vi "Get Config.vi"(0 "Sequence path":path=path "C:/ModisEdge/Scope/Test Sequence/ModisEdge.ini", 7 "File":string="ModisEdge.ini") -> (1 "Headers Path":path=path "C:/ModisEdge/Scope/Test Sequence/Headers_ModisEdge.ini", 2 "FixtureID":string="MEScope_Fixture1", 3 "StopTestOnFailure":bool=TRUE, 4 "StationID":string="TSNAFT202", 6 "Test Report Path":path=path "C:/Snap-On/ModisEdge_Scope", 8 "DAQ DEVICE NAME":string="Dev5", 10 "WriteTheHeaders":bool, 14 "UUT_COM":u32=5, 15 "error out":errorcluster)   [LabVIEW 2015]
uses:
  <vilib>/Utility/config.llb/Read Key (Boolean).vi
  <vilib>/Utility/config.llb/Read Key (String).vi
  <vilib>/Utility/config.llb/Read Key (Path).vi
  <vilib>/Utility/config.llb/Read Key (U32).vi
  <vilib>/Utility/config.llb/NI_LVConfig.lvlib
panel:
  out "appended path":path=path "C:/ModisEdge/Scope/Test Sequence/ModisEdge.ini"
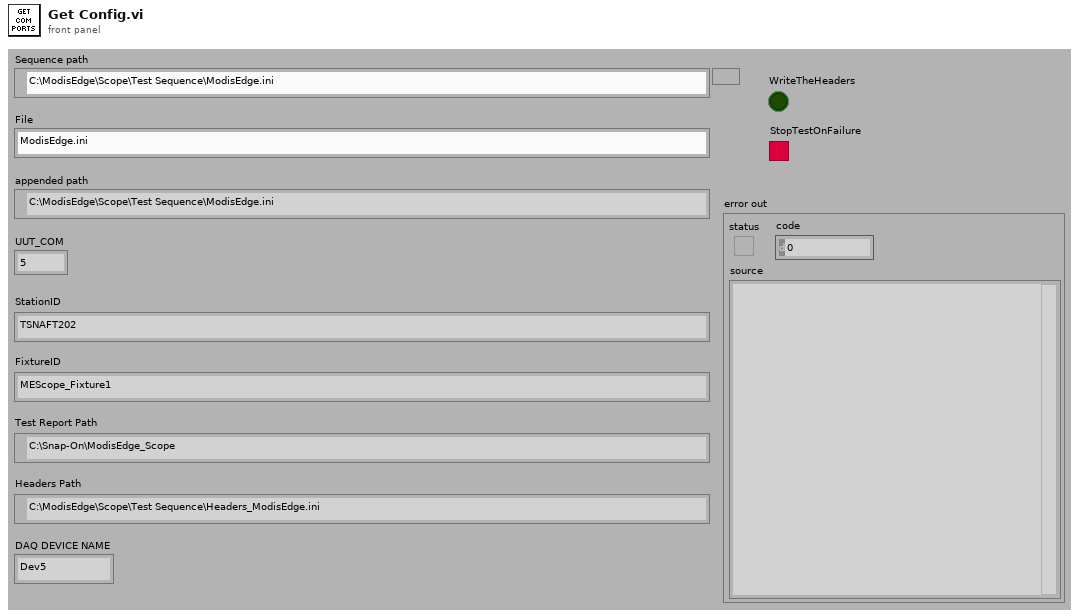
[diagram p1: front panel]
types:
  T1 = typedef "NI_LVConfig.lvlib/Config Data RefNum.ctl" = refnum<k1>
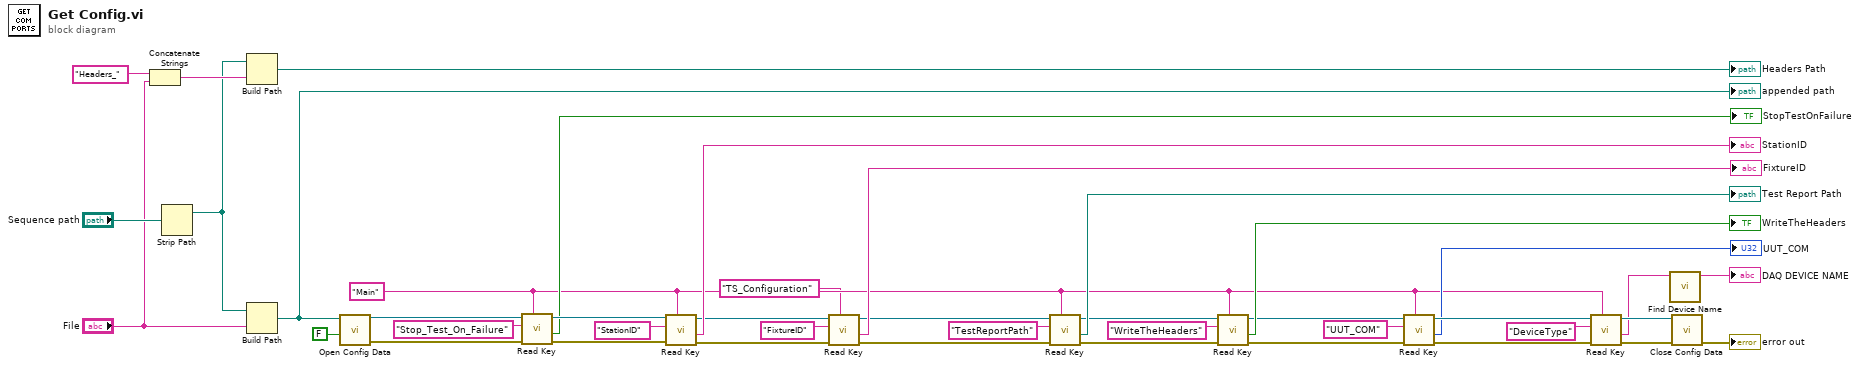
[diagram p0: block diagram]
diagram:
  w2 = "Main" ("section")
  n1 = Concatenate Strings("Headers_", "File") -> (w22:string)
  n2 = Strip Path(path="Sequence path") -> (stripped path=w21:path)  [unwired: 1 out]
  n3 = Build Path(base path=w21, name or relative path=w22) -> (appended path=→"Headers Path":path)
  n4 = Build Path(base path=w21, name or relative path="File") -> (appended path=w19:path)
  "appended path" <- w19
  n5 = call <vilib>:"Open Config Data.vi"("create file if necessary (T)"=FALSE, "configuration file path"=w19) -> ("error out"=w16:errorcluster, "refnum"=w17:T1)  [unwired: 7 in, 1 out]
  n6 = call-poly <vilib>:"Read Key.vi"("section"=w2, "error in (no error)"=w16, "key"="Stop_Test_On_Failure", "refnum"=w17) -> ("error out"=w15:errorcluster, "value"=→"StopTestOnFailure":bool, "refnum out"=w18:T1)  [unwired: 4 in, 1 out]
  n7 = call-poly <vilib>:"Read Key.vi"("section"=w2, "error in (no error)"=w15, "key"="StationID", "refnum"=w18) -> ("error out"=w7:errorcluster, "value"=→"StationID":string, "refnum out"=w3:T1)  [unwired: 4 in, 1 out]
  n8 = call-poly <vilib>:"Read Key.vi"("section"="TS_Configuration", "error in (no error)"=w7, "key"="FixtureID", "refnum"=w3) -> ("error out"=w6:errorcluster, "value"=→"FixtureID":string, "refnum out"=w4:T1)  [unwired: 4 in, 1 out]
  n9 = call-poly <vilib>:"Read Key.vi"("section"=w2, "error in (no error)"=w6, "key"="TestReportPath", "refnum"=w4) -> ("error out"=w34:errorcluster, "value"=→"Test Report Path":path, "refnum out"=w33:T1)  [unwired: 4 in, 1 out]
  n10 = call-poly <vilib>:"Read Key.vi"("section"=w2, "error in (no error)"=w34, "key"="WriteTheHeaders", "refnum"=w33) -> ("error out"=w28:errorcluster, "value"=→"WriteTheHeaders":bool, "refnum out"=w12:T1)  [unwired: 4 in, 1 out]
  n11 = call-poly <vilib>:"Read Key.vi"("section"=w2, "error in (no error)"=w28, "key"="UUT_COM", "refnum"=w12) -> ("error out"=w13:errorcluster, "value"=→"UUT_COM":u32, "refnum out"=w11:T1)  [unwired: 4 in, 1 out]
  n12 = call-poly <vilib>:"Read Key.vi"("section"=w2, "error in (no error)"=w13, "key"="DeviceType", "refnum"=w11) -> ("error out"=w27:errorcluster, "value"=w25:string, "refnum out"=w26:T1)  [unwired: 4 in, 1 out]
  n13 = call "Find Device Name.vi"("Device Type"=w25) -> ("Device Name"=→"DAQ DEVICE NAME":string)  [unwired: 10 in]
  n14 = call <vilib>:"Close Config Data.vi"("error in (no error)"=w27, "refnum"=w26) -> ("error out"=→"error out":errorcluster)  [unwired: 8 in, 1 out]
